vi "Read - Error Input - Returns Serialization Binder Base Class.vi"() -> ()   [LabVIEW 2017, in "Generic Object Serializer Tests.lvlib" / "Serialization Binder.lvlib"]
uses:
  Serialization Binder.lvlib
  Generic Object Serializer/Generic Object Serializer.lvclass
  Serialization Binder/Serialization Binder.lvclass
  Generic Object Serializer/Generic Object Serializer.lvclass/Generic Object Serializer.ctl
  Generic Object Serializer/Read Serialization Binder.vi
  Default Serialization Binder/Default Serialization Binder.lvclass
  C:/Users/de200256/Code/logmanoriginal/jsontext-object-serialization/Serialization Binder/Serialization Binder.lvclass
  <vilib>/Utility/error.llb/Error Cluster From Error Code.vi
  <vilib>/ErrorRing/Error Ring.xnode
  <vilib>/addons/_JKI Toolkits/Caraya/classes/Assert/Assert.lvclass
  <vilib>/addons/_JKI Toolkits/Caraya/classes/Test/Test.lvclass
panel:
  out "error out":errorcluster
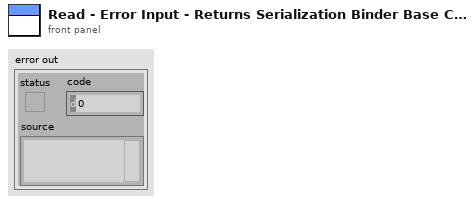
[diagram p1: front panel]
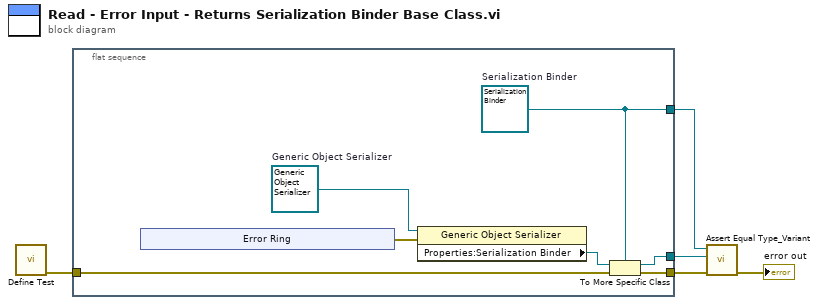
[diagram p0: block diagram]
diagram:
  n1 = call <vilib>:"Define Test.vi"() -> ("error out"=w3:errorcluster)  [unwired: 11 in]
  n2 = flat-sequence {
    tunnel: [w9] -> w5
    tunnel: [w8] -> w4
    tunnel: w3 -> [w7]
    tunnel: [w11] -> w2
    frame #0 {
      w8 = refnum<class "Serialization Binder.lvclass"> refnum  # Serialization Binder
      w12 = refnum<class "Generic Object Serializer.lvclass"> refnum  # Generic Object Serializer
      n3 = xnode "Error Ring"() -> ("error out"=w6:errorcluster)
      n4 = property class="Generic Object Serializer"(reference=w12, error in=w6) -> ("Properties:Serialization Binder"=w10:refnum<class "Serialization Binder.lvclass">)  [unwired: 2 out]
      n5 = To More Specific Class(target class=w8, reference=w10, error in=w7) -> (specific class reference=w9:refnum<class "Serialization Binder.lvclass">, error out=w11:errorcluster)
    }
  }
  n6 = call <vilib>:"Assert Equal Type_Variant.vi"("error in (no error)"=w2, "Y"=w5, "X"=w4) -> ("error out"=→"error out":errorcluster)  [unwired: 8 in]
